vi "Measurement Logic.vi"() -> ()   [LabVIEW 2024, in "Tone Generation.lvlib"]
uses:
  Tone Generation.lvlib
  <vilib>/Plug-In SDKs/Measurements/Measure Call Context/Measure Call Context.lvclass
  Measurement Configuration.ctl
  Measurement Results.ctl
  <vilib>/addons/_NISVFA/_Generation/Signal Generation/SV Signal/sv_System Timing Model.ctl
  <vilib>/DAQmx/write.llb/DAQmx Write (Analog 1D Wfm NChan NSamp).vi
  <extravilib>/ChannelInstances/Tag-bool/Read.vi
  <extravilib>/ChannelInstances/Tag-bool/Write.vi
  <extravilib>/ChannelInstances/Tag-bool/Read With Abort.vi
  <extravilib>/ChannelInstances/Tag-bool/Write With Abort.vi
  <vilib>/addons/_NISVFA/_Generation/Signal Generation/SV Sinusoid/SV Sinusoid.lvclass
  <extravilib>/ChannelInstances/Tag-bool/Instantiate.vi
  <vilib>/DAQmx/create/channels.llb/DAQmx Create Channel (AO-Voltage-Basic).vi
  <vilib>/DAQmx/configure/timing.llb/DAQmx Timing (Sample Clock).vi
  <vilib>/addons/_NISVFA/_Generation/Signal Generation/SV Signal/Write Sample Rate.vi
  <vilib>/addons/_NISVFA/_Generation/Signal Generation/SV Signal/Write System Timing Model.vi
  <vilib>/addons/_NISVFA/_Generation/Signal Generation/SV Signal/Write Ramp Parameters.vi
  <vilib>/addons/_NISVFA/_Generation/Signal Generation/SV Sinusoid/Configure Sine.vi
  <extravilib>/ChannelInstances/Tag-bool/EndpointRead.vi
  <extravilib>/ChannelInstances/Tag-bool/Endpoint.vi
  <vilib>/DAQmx/miscellaneous.llb/DAQmx Fill In Error Info.vi
  <extravilib>/ChannelInstances/Event Messenger-bool/Instantiate.vi
  <vilib>/addons/_NISVFA/_Generation/Signal Generation/SV Signal/SV Signal.lvclass
  <resource>/objmgr/daqmx.rc
panel:
  out "measurement results":T1={"error out"=FALSE, "error description out"="Empty", "error code out"=0}
  in  "measurement configuration":T2={"sample rate"=0.0, "physical channels"=["Lorem ipsum dolor sit", "Lorem ipsum dolor sit"], "ranges"=[32.0, 33.0], "terminal cfgs"=[0, 0], "frequencies"=[64.0, 65.0], "amplitudes"=[0.0, 0.0], "phases"=[-32.0, -33.0]}
  out "measure call context out":refnum<class "Measure Call Context.lvclass">
  in  "measure call context in":refnum<class "Measure Call Context.lvclass">
  out "error out":errorcluster
  in  "error in":errorcluster
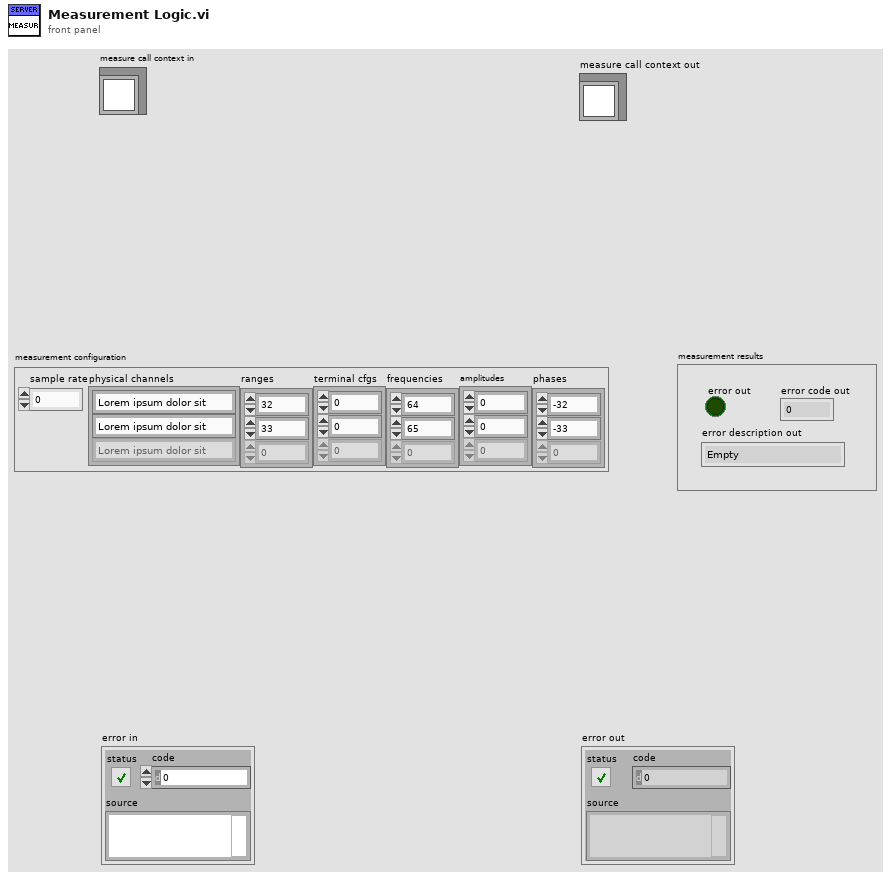
[diagram p1: front panel]
types:
  T1 = typedef "Tone Generation.lvlib/Measurement Results.ctl" = cluster{"error out":bool, "error description out":string, "error code out":i32}
  T2 = typedef "Tone Generation.lvlib/Measurement Configuration.ctl" = cluster{"sample rate":dbl, "physical channels":string[], "ranges":dbl[], "terminal cfgs":i32[], "frequencies":dbl[], "amplitudes":dbl[], "phases":dbl[]}
  T3 = cluster{"profile":enum16{"Linear", "Half cosine"}, "durations [s]":cluster{"ramp-up":dbl, "transition":dbl, "ramp-down":dbl}}
  T4 = typedef "SV Signal.lvclass/sv_System Timing Model.ctl" = i64
  T5 = typedef "Event Messenger-bool.lvlib/))Channel.ctl" = refnum<queue>
  T6 = typedef "Tag-bool.lvlib/))Channel.ctl" = refnum<queue>
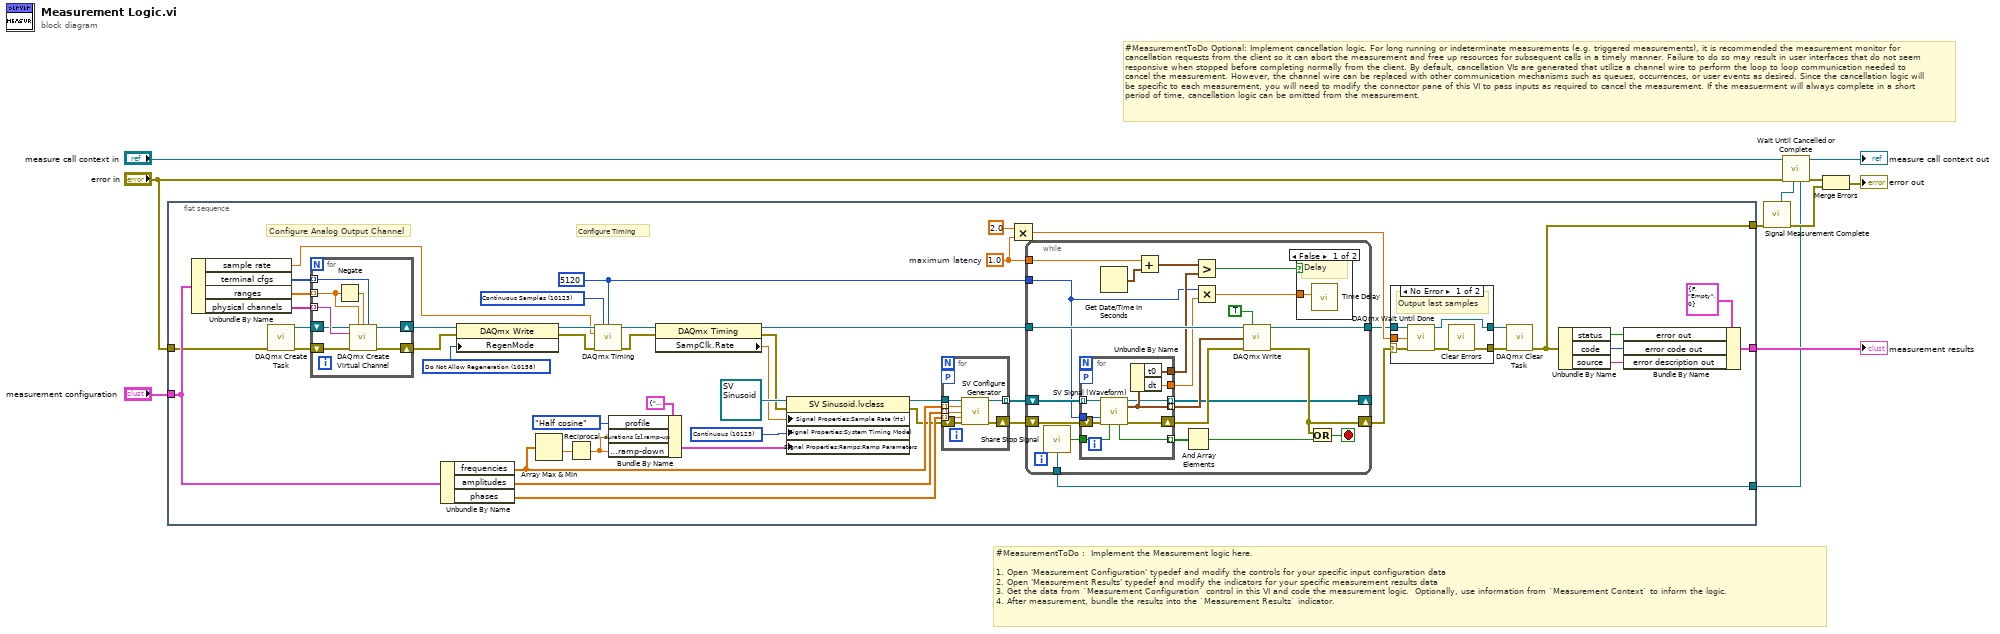
[diagram p0: block diagram]
diagram:
  # "#MeasurementToDo Optional: Implement cancellation logic. For long running or indeterminate measurements (e.g. triggered measurements), it is recommended the measurement monitor for cancellation requests from the client so it can abort the measurement and free up resources for subsequent calls in a timely manner. Failure to do so may result in user interfaces that do not seem responsive when stopped before completing normally from the client. By default, cancellation VIs are generated that utilize a channel wire to perform the loop to loop communication needed to cancel the measurement. However, the channel wire can be replaced with other communication mechanisms such as queues, occurrences, or user events as desired. Since the cancellation logic will be specific to each measurement, you will need to modify the connector pane of this VI to pass inputs as required to cancel the measurement. If the measuerment will always complete in a short period of time, cancellation logic can be omitted from the measurement."
  # "#MeasurementToDo :  Implement the Measurement logic here.\n\n1. Open 'Measurement Configuration' typedef and modify the controls for your specific input configuration data\n2. Open 'Measurement Results' typedef and modify the indicators for your specific measurement results data\n3. Get the data from `Measurement Configuration` control in this VI and code the measurement logic.  Optionally, use information from `Measurement Context` to inform the logic.\n4. After measurement, bundle the results into the `Measurement Results` indicator."
  n1 = flat-sequence {
    tunnel: "measurement configuration" -> [w53]
    tunnel: [w58] -> w10
    tunnel: "error in" -> [w18]
    tunnel: [w15] -> w6
    tunnel: w1 -> [w19]
    frame #0 {
      w30 = 10158 items=["Allow Regeneration"=10097, "Do Not Allow Regeneration"=10158] ("RegenMode")
      w13 = 5120 ("samples per channel")
      w39 = 10123 items=["Finite Samples"=10178, "Continuous Samples"=10123, "Hardware Timed Single Point"=12522] ("sample mode")
      w23 = 1.0  # maximum latency
      w55 = T4 10123 items=["Finite"=10178, "-"=-1, "Continuous"=10123, "-"=-2, "Settled"=110123, "Averaged"=210123, "Discrete Sweep"=310123, "Continuous Sweep"=410123] ("System Timing Model")
      # "Configure Timing"
      # "Configure Analog Output Channel"
      n2 = Unbundle By Name(w53) -> ("sample rate"=w17:dbl, "terminal cfgs"=w31:i32[], "ranges"=w32:dbl[], "physical channels"=w33:string[])
      n3 = call <vilib>:"DAQmx Create Task.vi"("error in"=w18) -> ("task out"=w29:refnum<k21>, "error out"=w28:errorcluster)  [unwired: 13 in]
      n4 = for {
        tunnel: w33 -> [w105] mode=indexing
        tunnel: w32 -> [w104] mode=indexing
        tunnel: w31 -> [w103] mode=indexing
        shift-right: [w107] -> w37
        shift-left: w29 -> [w102]
        shift-right: [w106] -> w35
        shift-left: w28 -> [w101]
        n5 = Negate(x=w104) -> (-x=w108:dbl)
        n6 = call-poly <vilib>:"DAQmx Create Virtual Channel.vi"("task in"=w102, "maximum value"=w104, "minimum value"=w108, "output terminal configuration"=w103, "physical channels"=w105, "error in"=w101) -> ("task out"=w107:refnum<k21>, "error out"=w106:errorcluster)  [unwired: 8 in]
      }
      n7 = Unbundle By Name(w53) -> ("frequencies"=w49:dbl[], "amplitudes"=w48:dbl[], "phases"=w47:dbl[])
      n8 = property class="DAQmx Write"(reference=w37, error in=w35, "RegenMode"=w30) -> (reference out=w36:refnum<k21>, error out=w34:errorcluster)
      n9 = Array Max & Min(array=w49) -> (min value=w54:dbl)  [unwired: 3 out]
      n10 = Reciprocal(x=w54) -> (1/x=w52:dbl)
      n11 = call-poly <vilib>:"DAQmx Timing.vi"("task/channels in"=w36, "sample mode"=w39, "samples per channel"=w13, "rate"=w17, "error in"=w34) -> ("task out"=w40:refnum<k21>, "error out"=w38:errorcluster)  [unwired: 9 in]
      n12 = Bundle By Name(cluster=T3 {"profile"=enum."Linear", "durations [s]"={"ramp-up"=0.0, "transition"=0.0, "ramp-down"=0.0}} ("Ramp Parameters:All Elements"), "profile"=enum16{"Linear", "Half cosine"}."Half cosine", "durations [s].ramp-up"=w52, "durations [s].ramp-down"=w52) -> (w56:T3)
      n13 = property class="DAQmx Timing"(reference=w40, error in=w38) -> (reference out=w22:refnum<k21>, error out=w26:errorcluster, "SampClk.Rate"=w27:dbl)
      n14 = property class="SV Sinusoid.lvclass"(reference=refnum<class "SV Sinusoid.lvclass"> refnum ("signal configuration"), error in=w26, "Signal Properties:Sample Rate (Hz)"=w27, "Signal Properties:System Timing Model"=w55, "Signal Properties:Ramps:Ramp Parameters"=w56) -> (reference out=w50:refnum<class "SV Sinusoid.lvclass">, error out=w46:errorcluster)
      n15 = for {
        tunnel: w50 -> [w115]
        tunnel: w49 -> [w114] mode=indexing
        tunnel: w48 -> [w113] mode=indexing
        tunnel: w47 -> [w112] mode=indexing
        tunnel: [w111] -> w45 mode=indexing
        workers-P: _ -> [_]
        shift-right: [w110] -> w44
        shift-left: w46 -> [w109]
        n16 = call-poly <vilib>:"SV Configure Generator.vi"("template configuration"=w115, "frequency (Hz)"=w114, "amplitude"=w113, "phase (deg)"=w112, "error in (no error)"=w109) -> ("signal configuration"=w111:refnum<class "SV Sinusoid.lvclass">, "error out"=w110:errorcluster)  [unwired: 9 in]
      }
      n17 = Multiply(x=2.0 ("value"), y=w23) -> (x*y=w24:dbl)
      n18 = while {
        tunnel: w23 -> [w63]
        tunnel: w22 -> [w77]
        shift-right: [w69] -> w20
        shift-left: w44 -> [w80]
        tunnel: [w74] -> w21
        tunnel: w19 -> [w73]
        shift-right: [w67] -> _
        shift-left: w45 -> [w81]
        tunnel: w13 -> [w60]
        stop <- w70 stop-if-true
        n19 = call <vilib>:"Share Stop Signal.vi"("channel"=w73) -> ("stop"=w72:bool)  [unwired: 1 in]
        n20 = for {
          tunnel: [w90] -> w78 mode=indexing
          workers-P: _ -> [_]
          tunnel: w81 -> [w92] mode=indexing
          tunnel: [w89] -> w61
          shift-right: [w88] -> w75
          shift-left: w80 -> [w91]
          tunnel: w72 -> [w87]
          tunnel: [w86] -> w71 mode=indexing
          tunnel: [w85] -> w67 mode=indexing
          tunnel: w60 -> [w84]
          tunnel: [w83] -> w66
          n21 = call-dynamic "SV Signal (Waveform).vi"("signal configuration"=w92, "samples"=w84, "error in (no error)"=w91, "stop"=w87) -> ("signal configuration"=w85:refnum<class "SV Sinusoid.lvclass">, "output waveform"=w90:waveform(dbl), "done"=w86:bool, "error out"=w88:errorcluster)  [unwired: 6 in, 2 out]
          n22 = Unbundle By Name(w90) -> ("t0"=w89:timestamp, "dt"=w83:dbl)
        }
        n23 = Get Date/Time In Seconds() -> (seconds since 1Jan1904=w64:timestamp)
        n24 = Add(x=w63, y=w64) -> (x+y=w62:timestamp)
        n25 = And Array Elements(Boolean array=w71) -> (logical AND=w68:bool)
        n26 = Greater?(x=w62, y=w61) -> (0:w79:bool)
        n27 = Multiply(x=w60, y=w66) -> (x*y=w65:dbl)
        n28 = call-poly <vilib>:"DAQmx Write.vi"("task/channels in"=w77, "auto start"=TRUE, "data"=w78, "error in"=w75) -> ("task out"=w74:refnum<k21>, "error out"=w69:errorcluster)  [unwired: 9 in, 1 out]
        n29 = case shown="False" w79 {
          tunnel: w65 -> [w82 _]
          frame False {
            # "Delay"
            n30 = call "Time Delay"("Delay Time (s)"=w82) -> ()  [unwired: 10 in, 1 out]
          }
          frame True {
            # "Continue"
          }
        }
        n31 = Or(x=w69, y=w68) -> (x .or. y?=w70:bool)
      }
      n32 = case shown="No Error" w20 {
        selector: w20 -> [w97 w100]
        tunnel: w21 -> [w98 w99]
        tunnel: w24 -> [w96 _]
        tunnel: [w95 w100] -> w16
        tunnel: [w93 w99] -> w14
        frame No Error {
          # "Output last samples"
          n33 = call <vilib>:"DAQmx Wait Until Done.vi"("task/channels in"=w98, "timeout (sec)"=w96, "error in"=w97) -> ("task out"=w93:refnum<k21>, "error out"=w94:errorcluster)  [unwired: 11 in]
          n34 = call <vilib>:"Clear Errors.vi"("error in (no error)"=w94) -> ("error out"=w95:errorcluster)  [unwired: 5 in, 1 out]
        }
        frame Error {
          # "Error"
        }
      }
      n35 = call <vilib>:"DAQmx Clear Task.vi"("task in"=w14, "error in"=w16) -> ("error out"=w15:errorcluster)  [unwired: 13 in]
      n36 = Unbundle By Name(w15) -> ("status"=w43:bool, "code"=w42:i32, "source"=w41:string)
      n37 = Bundle By Name(cluster=T1 {"error out"=FALSE, "error description out"="Empty", "error code out"=0} ("Measurement Results"), "error out"=w43, "error code out"=w42, "error description out"=w41) -> (w58:T1)
    }
  }
  n38 = call "Signal Measurement Complete.vi"("error in (no error)"=w6) -> ("error out"=w4:errorcluster, "done channel"=w5:T5)  [unwired: 9 in]
  n39 = call "Wait Until Cancelled or Complete.vi"("done channel"=w5, "error in (no error)"="error in", "measure call context in"="measure call context in") -> ("error out"=w3:errorcluster, "measure call context out"=→"measure call context out":refnum<class "Measure Call Context.lvclass">, "channel"=w1:T6)  [unwired: 6 in]
  n40 = Merge Errors(w3, w4) -> (→"error out":errorcluster)
  "measurement results" <- w10
